vi "GetBooleanValue.vi"(10 "true/false string":string) -> (2 "value":bool)   [LabVIEW 2014, in "Raspberry Pi Compatible Compiler for LabVIEW.lvlib" / "PythonConverter_GUI.lvclass"]
uses:
  PythonConverter_GUI.lvclass
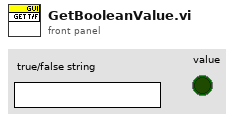
[diagram p1: front panel]
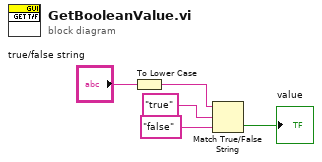
[diagram p0: block diagram]
diagram:
  n1 = To Lower Case(string="true/false string") -> (all lower case string=w5:string)
  n2 = Match True/False String(2:"false" ("false string"), 3:"true" ("true string"), 4:w5) -> (0:→"value":bool)  [unwired: 1 out]
